vi "VariableValue.vi"(10 "Value":dbl, 11 "Name":string) -> (3 "VariableValue":refnum<class "VariableValue.lvclass">)   [LabVIEW 2012, in "VariableManagerAPI.lvlib"]
doc: "Return Variable value object.\nThe object contains given values (optional).\nData can be accessed through property node.\n\n<B>Name</B>: The name of the value\n<B>Value</B>: The value of the name"
uses:
  VariableManagerAPI.lvlib
  VariableValue/VariableValue.lvclass
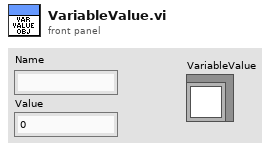
[diagram p1: front panel]
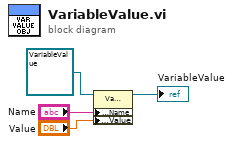
[diagram p0: block diagram]
diagram:
  n1 = property class="VariableValue.lvclass"(reference=refnum<class "VariableValue.lvclass"> refnum ("VariableValue.lvclass"), "Accessors:Name"="Name", "Accessors:Value"="Value") -> (reference out=→"VariableValue":refnum<class "VariableValue.lvclass">)  [unwired: 1 in, 1 out]
